vi "系统设置.vi"() -> (7 "簇":T1)   [LabVIEW 2021]
uses:
  <userlib>/_MGI/Timing/MGI Wait/MGI Wait (U32).vi
panel:
  in  "簇 2":T1
  in  "工况切换地址":refnum<visa-resource-name>
  in  "探头位置":u16(ring) items=["请选择", "111", "新建 文本文档"]
  in  "工况模式":enum16{"工况电流", "复合工况"}(ring)
  in  "大循环次数":dbl=1.0
  in  "工况2循环次数":dbl=1.0
  in  "工况2":u16(ring) items=["请选择", "111", "新建 文本文档"]
  in  "?":bool
  in  "扫描时间":dbl
  in  "测试总时间":dbl
  in  "工况1循环次数":dbl=1.0
  in  "工况1":u16(ring) items=["请选择", "111", "新建 文本文档"]
  in  "电流加载地址":refnum<visa-resource-name>
  in  "温度读取":refnum<visa-resource-name>
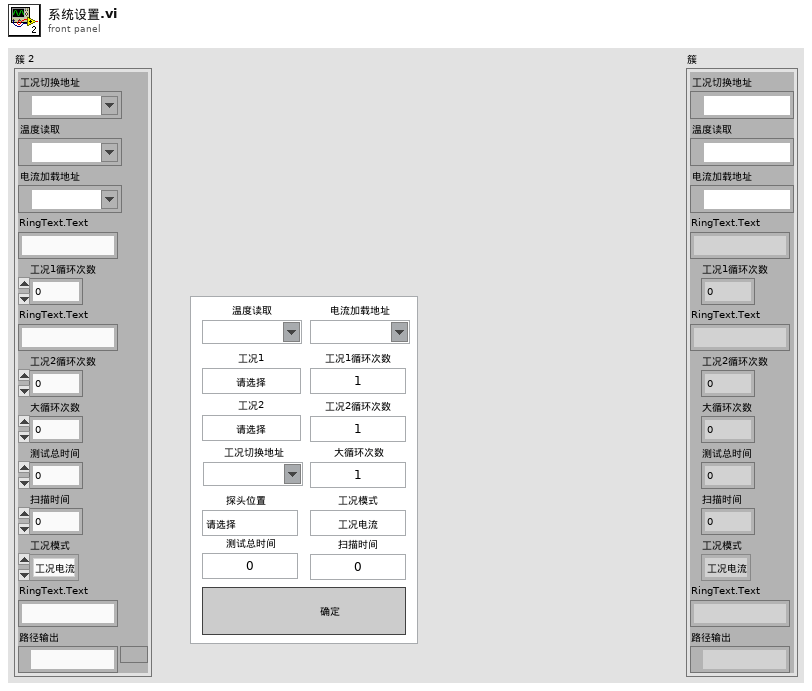
[diagram p1: front panel]
types:
  T1 = cluster{"工况切换地址":refnum<visa-resource-name>, "温度读取":refnum<visa-resource-name>, "电流加载地址":refnum<visa-resource-name>, "RingText.Text":string, "工况1循环次数":dbl, "RingText.Text":string, "工况2循环次数":dbl, "大循环次数":dbl, "测试总时间":dbl, "扫描时间":dbl, "工况模式":enum16{"工况电流", "复合工况"}, "RingText.Text":string, "路径输出":path}
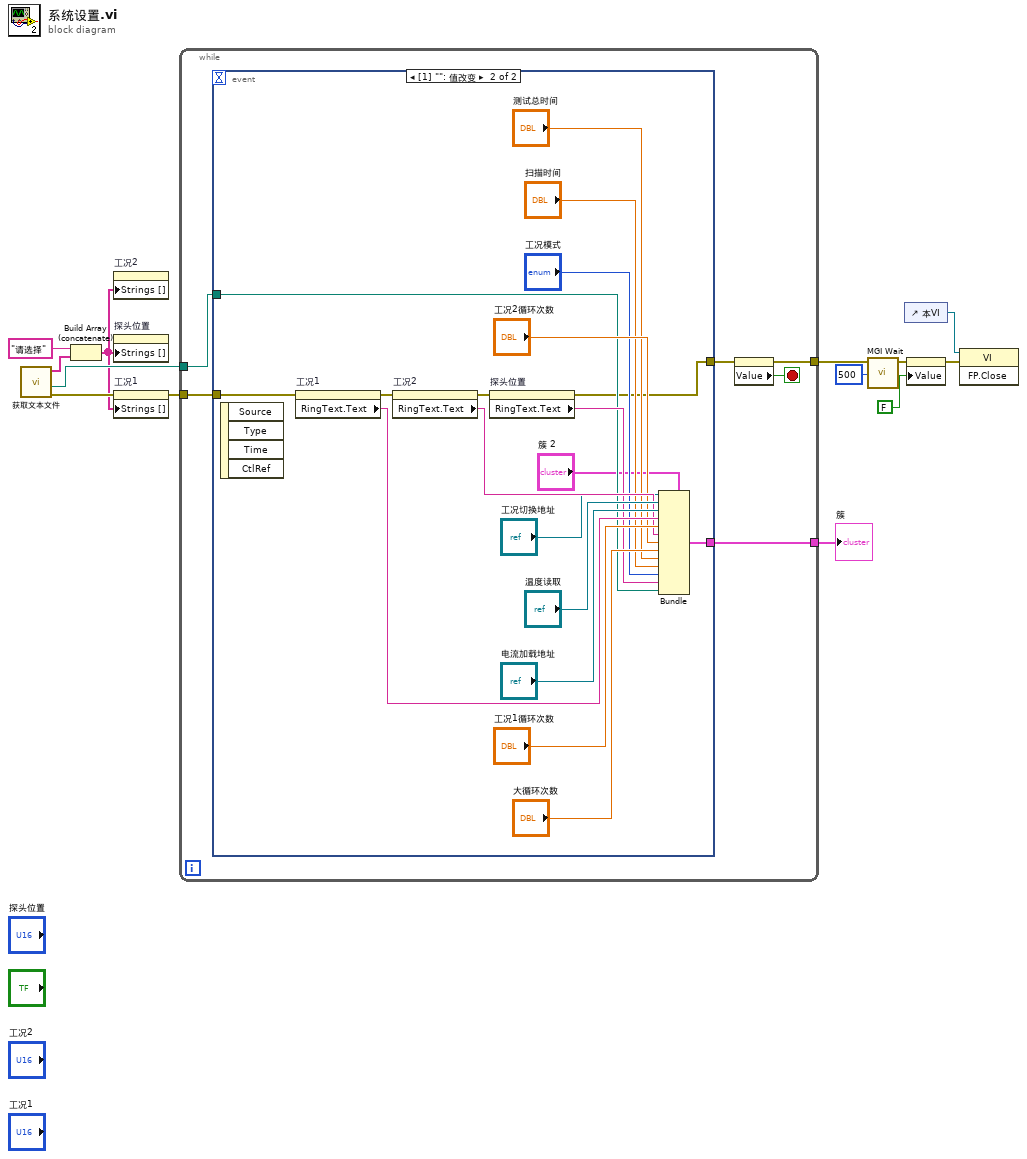
[diagram p0: block diagram]
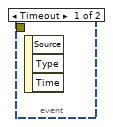
[diagram p2: hidden frame]
diagram:
  n1 = call "获取文本文件.vi"() -> ("错误输出"=w10:errorcluster, "路径输出"=w4:path, "数组"=w2:string[])  [unwired: 9 in]
  n2 = Build Array (concatenate)("请选择", w2) -> (w1:string[])
  n3 = property on="工况2" class="Ring (严格)"("Strings []"=w1) -> ()  [unwired: 2 in, 2 out]
  n4 = property on="探头位置" class="Ring (严格)"("Strings []"=w1) -> ()  [unwired: 2 in, 2 out]
  n5 = property on="工况1" class="Ring (严格)"(error in=w10, "Strings []"=w1) -> (error out=w9:errorcluster)  [unwired: 1 in, 1 out]
  n6 = while {
    tunnel: [w18] -> w12
    tunnel: w9 -> [w17]
    tunnel: [w16] -> w8
    tunnel: w4 -> [w15]
    stop <- w19 stop-if-true
    n7 = event shown="[1] \"\": 值改变" {
      selector: _ -> [_ _]
      dyn-events: _ -> [_ _]
      timeout: _ -> [_ _]
      tunnel: w17 -> [_ w36]
      tunnel: [_ w28] -> w16
      tunnel: w15 -> [_ w24]
      tunnel: [_ w20] -> w14
      event Timeout {
        n8 = event-data() -> ()  [unwired: 1 in, 3 out]
      }
      event Value Change {
        n9 = event-data() -> ()  [unwired: 1 in, 4 out]
        n10 = property on="工况1" class="Ring (严格)"(error in=w36) -> (error out=w22:errorcluster, "RingText.Text"=w35:string)  [unwired: 1 in, 1 out]
        n11 = property on="工况2" class="Ring (严格)"(error in=w22) -> (error out=w21:errorcluster, "RingText.Text"=w33:string)  [unwired: 1 in, 1 out]
        n12 = property on="探头位置" class="Ring (严格)"(error in=w21) -> (error out=w20:errorcluster, "RingText.Text"=w26:string)  [unwired: 1 in, 1 out]
        n13 = Bundle(cluster="簇 2", "工况切换地址"="工况切换地址", "温度读取"="温度读取", "电流加载地址"="电流加载地址", "RingText.Text"=w35, "工况1循环次数"="工况1循环次数", "RingText.Text"=w33, "工况2循环次数"="工况2循环次数", "大循环次数"="大循环次数", "测试总时间"="测试总时间", "扫描时间"="扫描时间", "工况模式"="工况模式", "RingText.Text"=w26, "路径输出"=w24) -> (w28:T1)
      }
    }
    n14 = property class="Bool (严格)"(error in=w14) -> (error out=w18:errorcluster, "Value"=w19:bool)  [unwired: 1 in, 1 out]
  }
  "簇" <- w8
  n15 = call-poly <userlib>:"MGI Wait.vi"("ms"=u32 500, "Error In"=w12) -> ("Error Out"=w6:errorcluster)  [unwired: 5 in]
  n16 = control-ref of="本VI"() -> (w13:refnum<vi>)
  n17 = property class="Bool (严格)"(error in=w6, "Value"=FALSE) -> (error out=w5:errorcluster)  [unwired: 1 in, 1 out]
  n18 = invoke class="VI" method="FP.Close"(reference=w13, error in=w5) -> ()  [unwired: 1 in, 3 out]
